vi "Tegam4040 - Coupling.vi"(0 "Instrument Session Handle In":u32 format="%x", 1 "Coupling":enum16{"DC Coupling", "AC Coupling"}(ring), 11 "error in (no error)":errorcluster) -> (4 "Instrument Session Handle Out (dupl)":u32 format="%x", 15 "error out":errorcluster)   [LabVIEW 2010, in "Tegam4040.lvlib"]
doc: "Coupling: This bit selects mode of input coupling.\n\n0: DC coupling (default)\n1: AC coupling"
uses:
  Tegam4040.lvlib
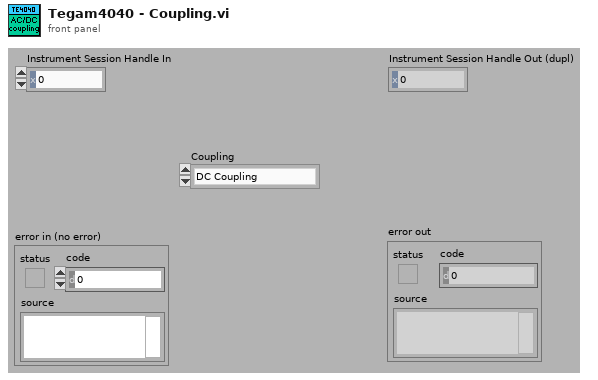
[diagram p1: front panel]
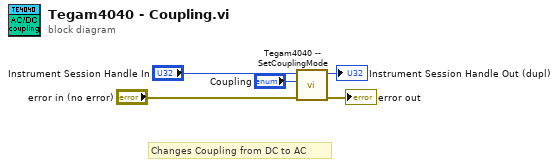
[diagram p0: block diagram]
diagram:
  # "Changes Coupling from DC to AC"
  n1 = call "Tegam4040 -- SetCouplingMode.vi"("error in (no error)"="error in (no error)", "Coupling"="Coupling", "Instrument Session Handle In"="Instrument Session Handle In") -> ("error out"=→"error out":errorcluster, "Instrument Session Handle Out (dupl)"=→"Instrument Session Handle Out (dupl)":u32)  [unwired: 7 in]
